vi "Calculate frame size and time.vi"(9 "AOD Fill time":dbl, 10 "Dwell Time":dbl, 11 "Patch Size":cluster{"X Length":i32, "Y Length":i32}) -> (0 "Frame Time (usec)":dbl, 1 "Y Length":i32, 2 "X Length":i32, 3 "Frame Time (ms)":dbl)   [LabVIEW 2020]
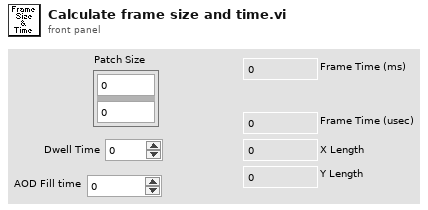
[diagram p1: front panel]
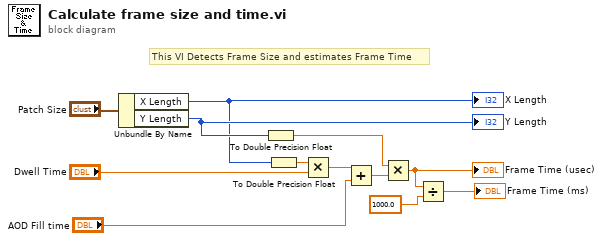
[diagram p0: block diagram]
diagram:
  # "This VI Detects Frame Size and estimates Frame Time"
  n1 = Unbundle By Name("Patch Size") -> ("X Length"=w1:i32, "Y Length"=w2:i32)
  "X Length" <- w1
  "Y Length" <- w2
  n2 = To Double Precision Float(number=w2) -> (double precision float=w7:dbl)
  n3 = To Double Precision Float(number=w1) -> (double precision float=w11:dbl)
  n4 = Multiply(x=w11, y="Dwell Time") -> (x*y=w10:dbl)
  n5 = Add(x=w10, y="AOD Fill time") -> (x+y=w8:dbl)
  n6 = Multiply(x=w7, y=w8) -> (x*y=w5:dbl)
  "Frame Time (usec)" <- w5
  n7 = Divide(x=w5, y=1000.0) -> (x/y=→"Frame Time (ms)":dbl)
